vi "AverageValue.vi"(2 "Running Input":dbl, 3 "N":dbl, 4 "Array In":dbl[](array[numeric])) -> (0 "Average":dbl, 1 "Array Out":dbl[](array[numeric]))   [LabVIEW 2021]
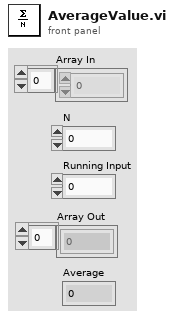
[diagram p1: front panel]
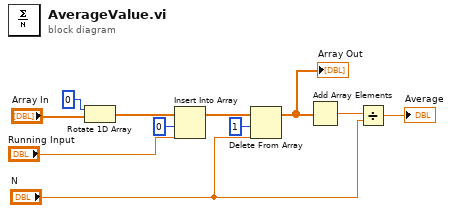
[diagram p0: block diagram]
diagram:
  n1 = Rotate 1D Array(1:"Array In", 2:0 ("n")) -> (0:w9:dbl[])
  n2 = Insert Into Array(array=w9, index=0, new element="Running Input") -> (w6:dbl[])
  n3 = Delete From Array(array=w6, length=1, index="N") -> (array with subset deleted=w1:dbl[])  [unwired: 1 out]
  "Array Out" <- w1
  n4 = Add Array Elements(numeric array=w1) -> (sum=w4:dbl)
  n5 = Divide(x=w4, y="N") -> (x/y=→"Average":dbl)
